vi "Verify Config Path.vi"(8 "error in (no error)":errorcluster, 11 "Config File Path":path) -> (0 "error out":errorcluster, 3 "Config File Path out":path)   [LabVIEW 2020, in "Base.lvclass"]
uses:
  Base.lvclass
  <vilib>/Utility/error.llb/Error Cluster From Error Code.vi
  <vilib>/ErrorRing/Error Ring.xnode
  Base.lvclass/Base.ctl
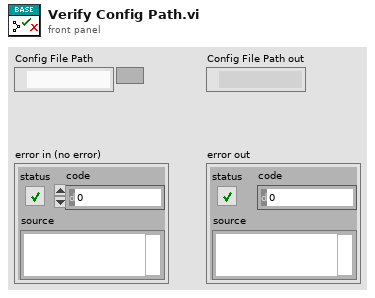
[diagram p1: front panel]
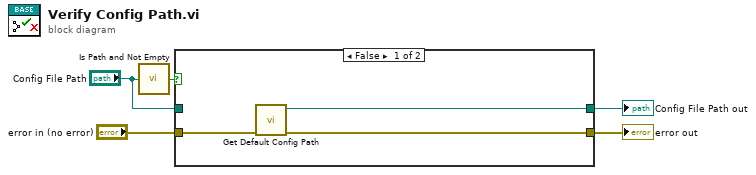
[diagram p0: block diagram]
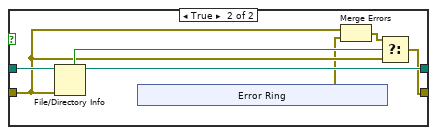
[diagram p2: hidden frame]
diagram:
  n1 = call <vilib>:"Is Path and Not Empty.vi"("path"="Config File Path") -> ("Is Path and Not Empty?"=w1:bool)  [unwired: 4 in]
  n2 = case shown="False" w1 {
    tunnel: "error in (no error)" -> [w8 w10]
    tunnel: [w7 w13] -> w5
    tunnel: [w6 w15] -> w4
    tunnel: "Config File Path" -> [_ w14]
    frame False {
      n3 = call "Get Default Config Path.vi"("error in (no error)"=w8) -> ("error out"=w7:errorcluster, "appended path"=w6:path)  [unwired: 9 in]
    }
    frame True {
      n4 = File/Directory Info(path=w14, error in=w10) -> (path out=w15:path, directory=w12:bool)  [unwired: 5 out]
      n5 = xnode "Error Ring"() -> ("error out"=w9:errorcluster)
      n6 = Merge Errors(w10, w9) -> (w11:errorcluster)
      n7 = Select(t=w11, s=w12, f=w10) -> (s? t:f=w13:errorcluster)
    }
  }
  "error out" <- w5
  "Config File Path out" <- w4
